vi "Write Pre-Addressed Publisher Messages.vi"(8 "Pre-Addressed Unlock Publication Msg":refnum<class "Unlock Publication Msg.lvclass">, 9 "Pre-Addressed Lock Publication Msg":refnum<class "Lock Publication Msg.lvclass">, 10 "Pre-Addressed Publish Msg":refnum<class "Publish Msg.lvclass">, 11 "IModel in":refnum<class "IModel.lvclass">) -> (3 "IModel out":refnum<class "IModel.lvclass">)   [LabVIEW 2020, in "IModel.lvlib" / "IModel.lvclass"]
doc: "写入预先写好地址的发布者消息"
uses:
  IModel.lvclass
  IMediator/IMediator Messages/Publish Msg/Publish Msg.lvclass
  IMediator/IMediator Messages/Lock Publication Msg/Lock Publication Msg.lvclass
  IMediator/IMediator Messages/Unlock Publication Msg/Unlock Publication Msg.lvclass
  IModel.lvclass/IModel.ctl
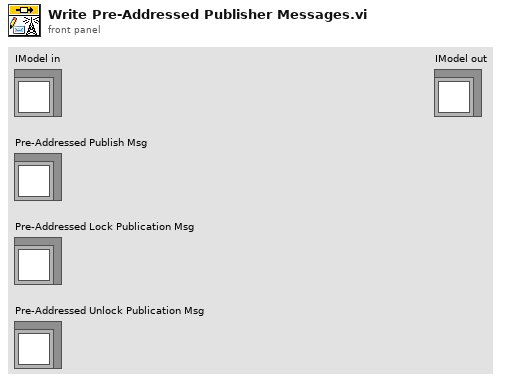
[diagram p1: front panel]
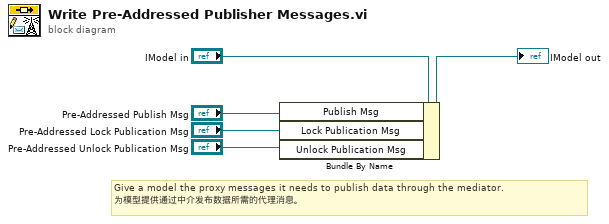
[diagram p0: block diagram]
diagram:
  # "Give a model the proxy messages it needs to publish data through the mediator.\n为模型提供通过中介发布数据所需的代理消息。"
  n1 = Bundle By Name(cluster="IModel in", "Publish Msg"="Pre-Addressed Publish Msg", "Lock Publication Msg"="Pre-Addressed Lock Publication Msg", "Unlock Publication Msg"="Pre-Addressed Unlock Publication Msg") -> (→"IModel out":refnum<class "IModel.lvclass">)
